vi "Log_ADAM_scan_table.vi"() -> ()   [LabVIEW 2015]
uses:
  ADAM Client/Sub VIs/ADAM Controls/Channel_State.ctl
  Anemometry/Anemometry Sub Vis/Globals/Constants_global.vi
  Anemometry/Anemometry Sub Vis/Globals/Preference_global.vi
  ADAM_Global.vi
  Anemometry/Anemometry Sub Vis/Globals/Meas_global.vi
panel:
  in  "High Res Day files":bool=TRUE
  in  "Ventilate Lab if temp above":dbl=21.5
  in  "Averaging time (Seconds)":dbl=60.0
  out "Current time":string
  out "Started Time":string
  in  "stop":bool
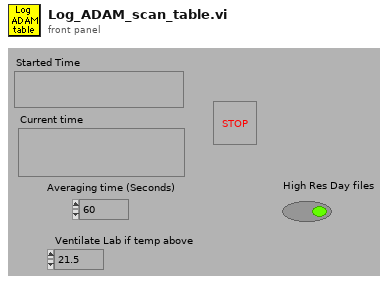
[diagram p1: front panel]
types:
  T1 = enum16{"On", "Off", "Always On", "Always Off", "Delete"}
  T2 = typedef "Channel_State.ctl" = enum16{"On", "Off", "Always On", "Always Off"}
  T3 = enum16{"Load ADAM setup from excel file", "Save ADAM setup to excel file"}
  T4 = cluster{"second":i32, "minute":i32, "hour":i32, "day of month":i32, "month":i32, "year":i32, "day of week":i32, "day of year":i32, "is DST":i32}
  T5 = typedef "Client_State_Cluster.ctl" = cluster{"Client Name":string, "Traverse level State":T6, "People to Email":string[], "Next Contact Time":dbl}
  T6 = typedef "Traverse_Level_State.ctl" = enum16{"Running", "Complete"}
  T7 = typedef "Server_Control.ctl" = cluster{"Channel Name to control":string, "Channel sharing":enum16{"Channel Unshared", "Channel Shared by Rig", "Channel Shared by Group"}, "Default Value":dbl, "Client Array":string[], "Time Stamp":timestamp, "Do Not Reset":bool}
  T8 = typedef "LVDateTimeRec.ctl" = cluster{"fractional second":dbl, "second":i32, "minute":i32, "hour":i32, "day of month":i32, "month":i32, "year":i32, "day of week":i32, "day of year":i32, "DST":i32}
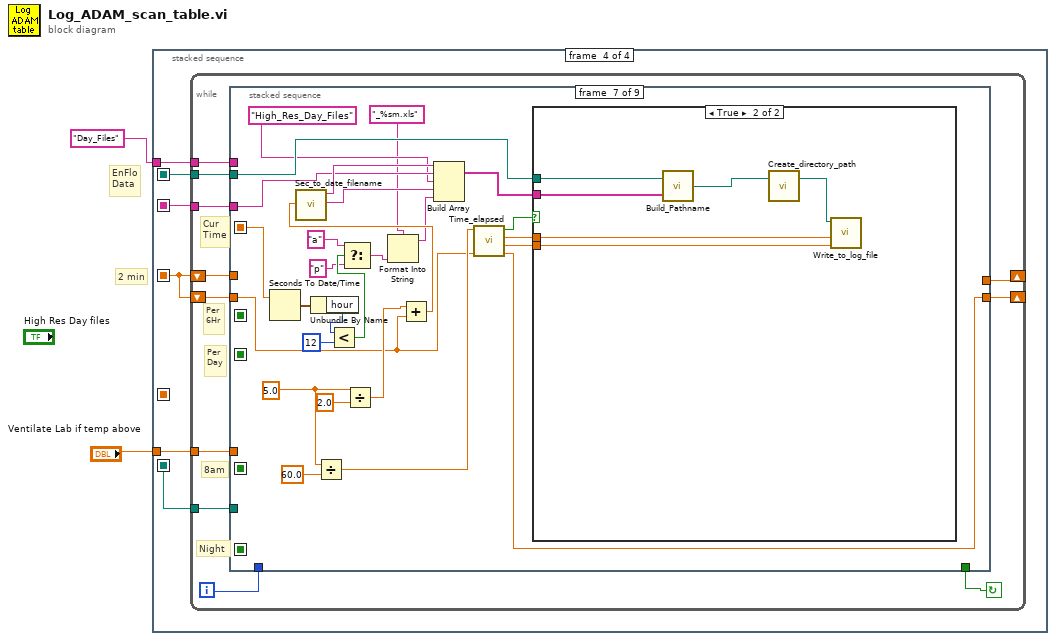
[diagram p0: block diagram]
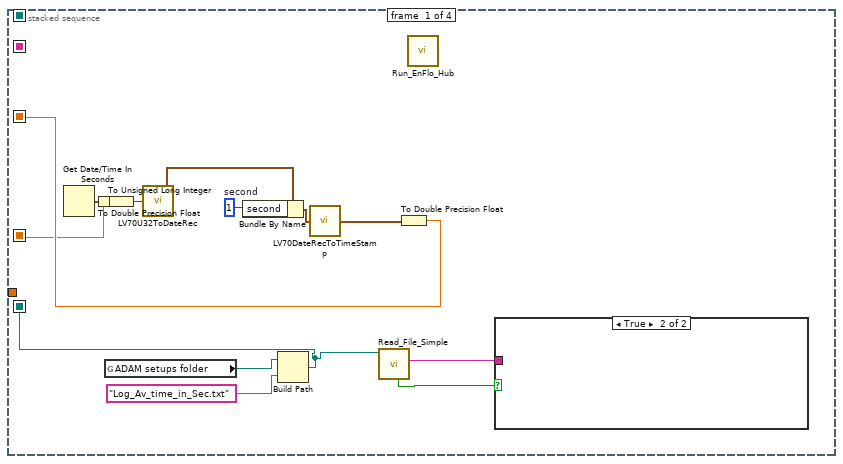
[diagram p2: hidden frame]
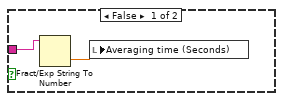
[diagram p3: hidden frame]
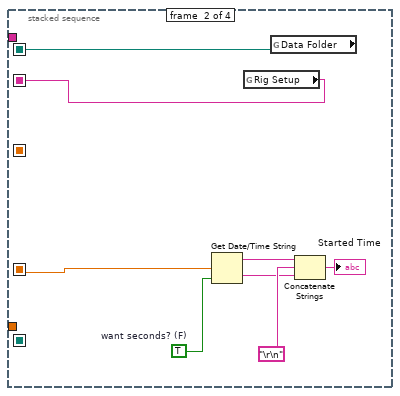
[diagram p4: hidden frame]
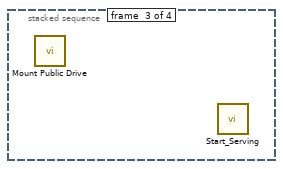
[diagram p5: hidden frame]
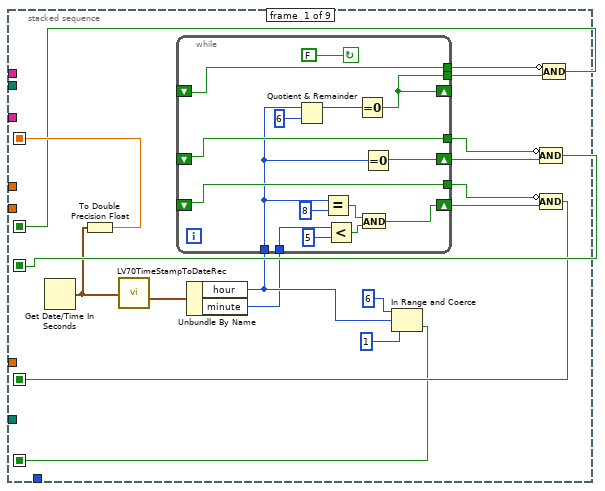
[diagram p6: hidden frame]
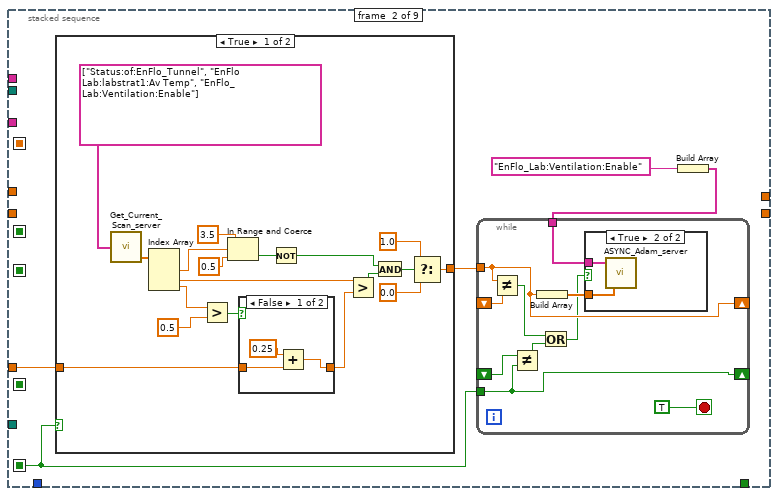
[diagram p7: hidden frame]
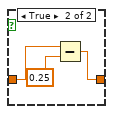
[diagram p9: hidden frame]
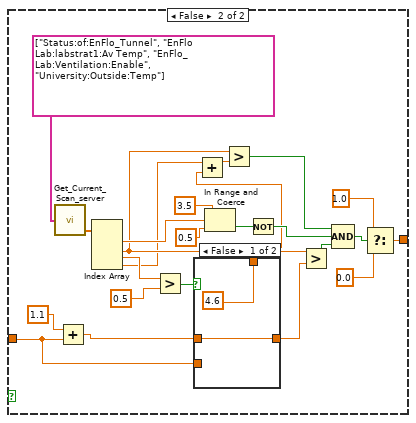
[diagram p10: hidden frame]
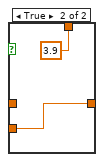
[diagram p11: hidden frame]
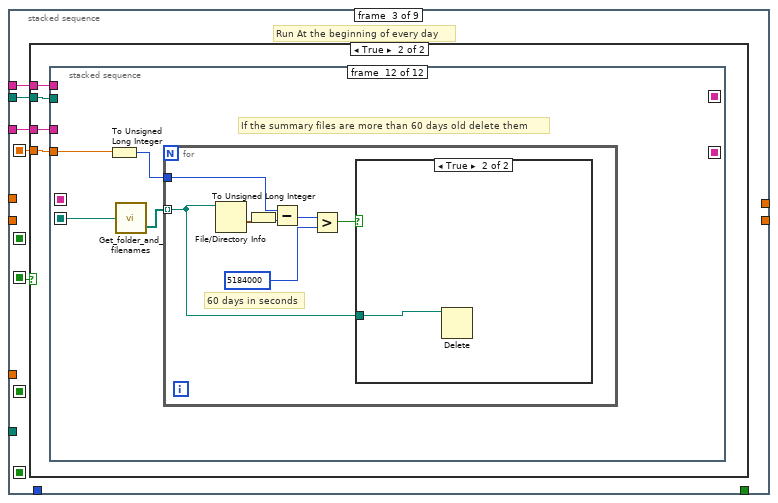
[diagram p12: hidden frame]
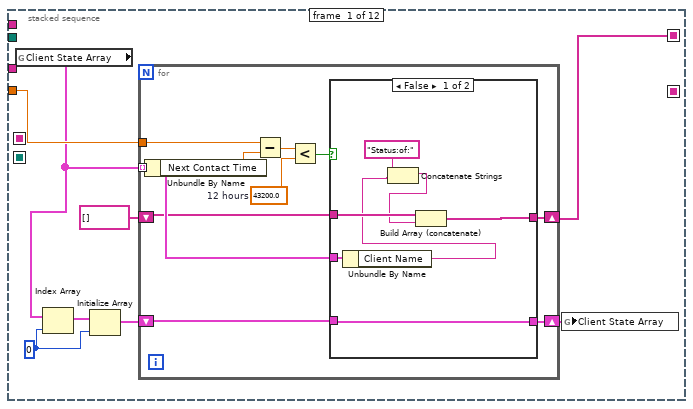
[diagram p14: hidden frame]
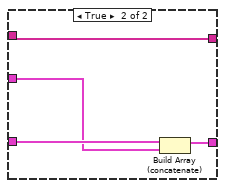
[diagram p15: hidden frame]
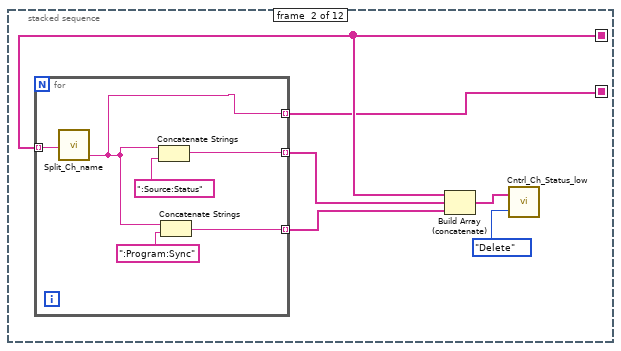
[diagram p16: hidden frame]
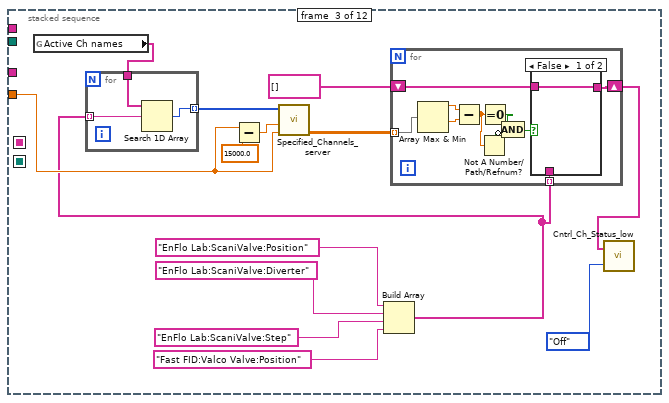
[diagram p17: hidden frame]
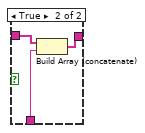
[diagram p18: hidden frame]
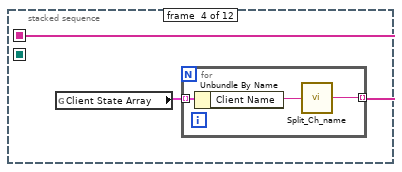
[diagram p19: hidden frame]
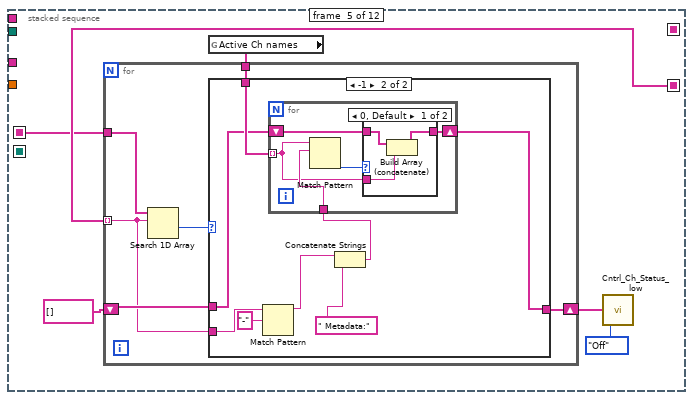
[diagram p20: hidden frame]
diagram:
  # "EnFlo\nData"
  # "2 min"
  n1 = stacked-sequence {
    seq-local: [w13 _ _ _] -> [_ _ _ w26]
    seq-local: [w12 _ _ _] -> [_ w25 _ _]
    seq-local: [_ w19 _ _] -> [_ _ _ w31]
    seq-local: [w5 _ _ _] -> [_ _ _ w29]
    seq-local: [_ w18 _ _] -> [_ _ _ w28]
    tunnel: "Day_Files" ("Input Element") -> [_ _ _ w30]
    tunnel: "Ventilate Lab if temp above" -> [_ _ _ w27]
    frame #0 {
      w15 = 1  # second
      n2 = Get Date/Time In Seconds() -> (seconds since 1Jan1904=w9:timestamp)
      n3 = To Double Precision Float(number=w9) -> (double precision float=w12:dbl)
      n4 = global read "Constants_global.vi" "ADAM setups folder"() -> (w7:path)
      n5 = To Unsigned Long Integer(number=w12) -> (unsigned 32bit integer=w11:u32)
      n6 = call <vilib>:"LV70U32ToDateRec.vi"("Time"=w11) -> ("date time rec"=w10:T4)
      n7 = Bundle By Name(cluster=w10, "second"=w15) -> (w14:T4)
      n8 = Build Path(base path=w7, name or relative path="Log_Av_time_in_Sec.txt") -> (appended path=w5:path)
      n9 = call <vilib>:"LV70DateRecToTimeStamp.vi"("date time rec"=w14) -> ("Time Stamp"=w8:timestamp)
      n10 = call "Read_File_Simple.vi"("Filename"=w5) -> ("Error?"=w3:bool, "string"=w4:string)  [unwired: 2 in, 6 out]
      n11 = To Double Precision Float(number=w8) -> (double precision float=w13:dbl)
      n12 = call "Run_EnFlo_Hub.vi"() -> ()  [unwired: 8 out]
      n13 = case shown="True" w3 {
        tunnel: w4 -> [w17 _]
        frame False {
          n14 = Fract/Exp String To Number(string=w17) -> (number=w16:dbl)  [unwired: 4 out]
          n15 = local write "Averaging time (Seconds)"(w16) -> ()
        }
        frame True {
        }
      }
    }
    frame #1 {
      w24 = TRUE  # want seconds? (F)
      n16 = Get Date/Time String(seconds (now)=w25, want seconds? (F)=w24) -> (date string=w22:string, time string=w21:string)  [unwired: 1 out]
      n17 = global read "Preference_global.vi" "Rig Setup"() -> (w18:string)
      n18 = global read "Constants_global.vi" "Data Folder"() -> (w19:path)
      n19 = Concatenate Strings(w22, "\r\n", w21) -> (→"Started Time":string)
    }
    frame #2 {
      n20 = call "Mount Public Drive.vi"() -> ()  [unwired: 12 in]
      n21 = call "Start_Serving.vi"() -> ()  [unwired: 1 out]
    }
    frame #3 {
      n22 = while {
        tunnel: w31 -> [w40]
        shift-left: w26 -> [w42]
        shift-right: [w41] -> _
        tunnel: w30 -> [w37]
        tunnel: w29 -> [w36]
        tunnel: w28 -> [w35]
        tunnel: w27 -> [w34]
        shift-right: [w32] -> _
        shift-left: w26 -> [w33]
        i -> [w39]
        stop <- w38 continue-if-true
        # "Night"
        # "8am"
        # "Per\n6Hr"
        # "Per\nDay"
        # "Cur\nTime"
        n23 = stacked-sequence {
          seq-local: [w52 _ _ _ _ _ _ _ _] -> [_ _ w148 _ _ _ _ _ _]
          seq-local: [w58 _ _ _ _ _ _ _ _] -> [_ _ w147 w374 w393 _ w433 _ _]
          seq-local: [w55 _ _ _ _ _ _ _ _] -> [_ _ _ _ _ _ _ _ _]
          seq-local: [w48 _ _ _ _ _ _ _ _] -> [_ _ _ w370 _ _ _ _ _]
          seq-local: [w44 _ _ _ _ _ _ _ _] -> [_ w75 _ _ _ _ _ _ _]
          tunnel: [_ _ _ _ _ w400 _ _ _] -> w41
          tunnel: w42 -> [_ _ _ _ _ w401 _ _ _]
          tunnel: w40 -> [_ _ w146 w373 _ w408 w448 _ _]
          tunnel: w39 -> [_ _ _ _ _ _ _ _ _]
          tunnel: [_ _ _ _ _ _ _ _ w468] -> w38
          tunnel: w37 -> [_ _ w145 w372 _ w398 _ _ _]
          tunnel: w36 -> [_ _ _ _ _ _ _ _ w467]
          tunnel: w35 -> [_ _ w144 w371 _ w402 w443 _ _]
          tunnel: w34 -> [_ w76 _ _ _ _ _ _ _]
          tunnel: w33 -> [_ _ _ _ _ _ w441 _ _]
          tunnel: [_ _ _ _ _ _ w440 _ _] -> w32
          frame #0 {
            n24 = Get Date/Time In Seconds() -> (seconds since 1Jan1904=w51:timestamp)
            n25 = To Double Precision Float(number=w51) -> (double precision float=w58:dbl)
            n26 = call <vilib>:"LV70TimeStampToDateRec.vi"("time stamp"=w51) -> ("date time rec"=w59:T4)
            n27 = Unbundle By Name(w59) -> ("hour"=w47:i32, "minute"=w43:i32)
            n28 = while {
              tunnel: [w69] -> w53
              shift-left: _ -> [w69]
              shift-right: [w70] -> w54
              tunnel: [w71] -> w56
              tunnel: [w72] -> w57
              tunnel: w47 -> [w66]
              shift-left: _ -> [w71]
              shift-right: [w72] -> _
              tunnel: [w67] -> w50
              shift-right: [w60] -> w49
              shift-left: _ -> [w67]
              tunnel: w43 -> [w64]
              stop <- FALSE continue-if-true
              n29 = Quotient & Remainder(x=w66, y=6) -> (x-y*floor(x/y)=w73:i32)  [unwired: 1 out]
              n30 = Equal?(x=w66, y=8) -> (x = y?=w61:bool)
              n31 = Less?(x=w64, y=5) -> (x < y?=w62:bool)
              n32 = Equal To 0?(x=w73) -> (x = 0?=w72:bool)
              n33 = And(x=w61, y=w62) -> (x .and. y?=w60:bool)
              n34 = Equal To 0?(x=w66) -> (x = 0?=w70:bool)
            }
            n35 = In Range and Coerce(upper limit=6, x=w47, lower limit=1) -> (In Range?=w44:bool)  [unwired: 1 out]
            n36 = Compound Arithmetic op=AND(invert w53, w54) -> (w52:bool)
            n37 = Compound Arithmetic op=AND(invert w50, w49) -> (w48:bool)
            n38 = Compound Arithmetic op=AND(invert w56, w57) -> (w55:bool)
          }
          frame #1 {
            n39 = case shown="True" w75 {
              tunnel: [w102 w133] -> w77
              tunnel: w76 -> [w92 w116]
              frame True {
                n40 = call "Get_Current_Scan_server.vi"("Desired Channels"=string[] ["Status:of:EnFlo_Tunnel", "EnFlo Lab:labstrat1:Av Temp", "EnFlo_Lab:Ventilation:Enable"]) -> ("Numerical Values"=w108:dbl[])  [unwired: 2 out]
                n41 = Index Array(array=w108) -> (element #1=w101:dbl, element #2=w107:dbl, element #3=w96:dbl)  [unwired: 3 in]
                n42 = Greater?(x=w96, y=0.5) -> (0:w94:bool)
                n43 = In Range and Coerce(upper limit=3.5, x=w101, lower limit=0.5) -> (In Range?=w98:bool)  [unwired: 1 out]
                n44 = case shown="False" w94 {
                  tunnel: [w111 w113] -> w93
                  tunnel: w92 -> [w112 w115]
                  frame False {
                    n45 = Add(x=0.25, y=w112) -> (x+y=w111:dbl)
                  }
                  frame True {
                    n46 = Subtract(x=w115, y=0.25) -> (x-y=w113:dbl)
                  }
                }
                n47 = Not(x=w98) -> (.not. x?=w97:bool)
                n48 = Greater?(x=w107, y=w93) -> (0:w106:bool)
                n49 = And(x=w97, y=w106) -> (x .and. y?=w105:bool)
                n50 = Select(t=1.0, s=w105, f=0.0) -> (s? t:f=w102:dbl)
              }
              frame False {
                n51 = call "Get_Current_Scan_server.vi"("Desired Channels"=string[] ["Status:of:EnFlo_Tunnel", "EnFlo Lab:labstrat1:Av Temp", "EnFlo_Lab:Ventilation:Enable", "University:Outside:Temp"]) -> ("Numerical Values"=w138:dbl[])  [unwired: 2 out]
                n52 = Add(x=1.1, y=w116) -> (x+y=w123:dbl)
                n53 = Index Array(array=w138) -> (element #1=w132:dbl, element #2=w121:dbl, element #3=w127:dbl, element #4=w120:dbl)  [unwired: 4 in]
                n54 = Greater?(x=w127, y=0.5) -> (0:w125:bool)
                n55 = case shown="False" w125 {
                  tunnel: [w141 w142] -> w124
                  tunnel: w123 -> [w141 _]
                  tunnel: [4.6 ("y") 3.9 ("y")] -> w117
                  tunnel: w116 -> [_ w142]
                  frame False {
                  }
                  frame True {
                  }
                }
                n56 = Add(x=w120, y=w117) -> (x+y=w119:dbl)
                n57 = In Range and Coerce(upper limit=3.5, x=w132, lower limit=0.5) -> (In Range?=w129:bool)  [unwired: 1 out]
                n58 = Greater?(x=w121, y=w119) -> (0:w118:bool)
                n59 = Not(x=w129) -> (.not. x?=w128:bool)
                n60 = Greater?(x=w121, y=w124) -> (0:w137:bool)
                n61 = Compound Arithmetic op=AND(w118, w128, w137) -> (w136:bool)
                n62 = Select(t=1.0, s=w136, f=0.0) -> (s? t:f=w133:dbl)
              }
            }
            n63 = Build Array("EnFlo_Lab:Ventilation:Enable") -> (w78:string[])
            n64 = while {
              shift-right: [w87] -> _
              shift-left: _ -> [w88]
              tunnel: w77 -> [w87]
              tunnel: w78 -> [w85]
              shift-right: [w84] -> _
              shift-left: _ -> [w83]
              tunnel: w75 -> [w84]
              stop <- TRUE stop-if-true
              n65 = Not Equal?(x=w87, y=w88) -> (x != y?=w81:bool)
              n66 = Not Equal?(x=w83, y=w84) -> (x != y?=w82:bool)
              n67 = Build Array(w87) -> (w89:dbl[])
              n68 = Or(x=w81, y=w82) -> (x .or. y?=w80:bool)
              n69 = case shown="True" w80 {
                tunnel: w89 -> [_ w91]
                tunnel: w85 -> [_ w90]
                frame False {
                }
                frame True {
                  n70 = call "ASYNC_Adam_server.vi"("Values"=w91, "Channel Names"=w90) -> ()  [unwired: 1 in, 3 out]
                }
              }
            }
          }
          frame #2 {
            # "Run At the beginning of every day"
            n71 = case shown="True" w148 {
              tunnel: w147 -> [_ w152]
              tunnel: w146 -> [_ w151]
              tunnel: w145 -> [_ w150]
              tunnel: w144 -> [_ w149]
              frame False {
              }
              frame True {
                n72 = stacked-sequence {
                  seq-local: [w153 _ _ _ _ _ _ _ _ _ _ _] -> [_ w187 _ _ _ _ _ _ w307 _ _ _]
                  seq-local: [_ w183 _ _ _ _ _ _ _ _ _ _] -> [_ _ _ _ w235 _ _ _ _ _ _ _]
                  seq-local: [_ _ _ w225 _ _ _ _ _ _ _ _] -> [_ _ _ _ w232 _ _ _ _ _ _ _]
                  seq-local: [_ _ _ _ _ _ _ _ _ _ w356 _] -> [_ _ _ _ _ _ _ _ _ _ _ w360]
                  tunnel: w152 -> [w160 _ w204 _ _ _ _ _ _ w354 _ w361]
                  tunnel: w151 -> [_ _ _ _ _ _ _ _ _ _ _ _]
                  tunnel: w150 -> [_ _ _ _ _ _ _ _ _ _ _ _]
                  tunnel: w149 -> [_ _ _ _ _ _ _ _ _ _ _ _]
                  frame #0 {
                    w158 = 0 ("Index")
                    n73 = global read "ADAM_Global.vi" "Client State Array"() -> (w159:T5[])
                    n74 = Index Array(array=w159, index=w158) -> (element=w157:T5)
                    n75 = Initialize Array(w157, w158) -> (w156:T5[])
                    n76 = for {
                      tunnel: w159 -> [w163] mode=indexing
                      shift-right: [w164] -> w155
                      shift-left: w156 -> [w165]
                      tunnel: w160 -> [w170]
                      shift-right: [w161] -> w153
                      shift-left: string[] [] -> [w162]
                      w167 = 43200.0  # 12 hours
                      n77 = Unbundle By Name(w163) -> ("Next Contact Time"=w169:dbl)
                      n78 = Subtract(x=w170, y=w169) -> (x-y=w168:dbl)
                      n79 = Less?(x=w168, y=w167) -> (x < y?=w166:bool)
                      n80 = case shown="False" w166 {
                        tunnel: w165 -> [w177 w181]
                        tunnel: [w177 w180] -> w164
                        tunnel: w163 -> [w176 w179]
                        tunnel: w162 -> [w175 w178]
                        tunnel: [w174 w178] -> w161
                        frame False {
                          n81 = Unbundle By Name(w176) -> ("Client Name"=w172:string)
                          n82 = Concatenate Strings("Status:of:", w172) -> (w171:string)
                          n83 = Build Array (concatenate)(w175, w171) -> (w174:string[])
                        }
                        frame True {
                          n84 = Build Array (concatenate)(w181, w179) -> (w180:T5[])
                        }
                      }
                    }
                    n85 = global write "ADAM_Global.vi" "Client State Array"(w155) -> ()
                  }
                  frame #1 {
                    n86 = for {
                      tunnel: w187 -> [w193] mode=indexing
                      tunnel: [w190] -> w185 mode=indexing
                      tunnel: [w189] -> w184 mode=indexing
                      tunnel: [w188] -> w183 mode=indexing
                      n87 = call "Split_Ch_name.vi"("Ch name"=w193) -> ("Low level"=w188:string)  [unwired: 2 out]
                      n88 = Concatenate Strings(w188, ":Source:Status") -> (w190:string)
                      n89 = Concatenate Strings(w188, ":Program:Sync") -> (w189:string)
                    }
                    n90 = Build Array (concatenate)(w187, w185, w184) -> (w186:string[])
                    n91 = call "Cntrl_Ch_Status_low.vi"("Mode"=T1."Delete", "Channel names"=w186) -> ()  [unwired: 1 out]
                  }
                  frame #2 {
                    n92 = global read "ADAM_Global.vi" "Active Ch names"() -> (w207:string[])
                    n93 = Subtract(x=w204, y=15000.0) -> (x-y=w202:dbl)
                    n94 = Build Array("EnFlo Lab:ScaniValve:Position", "EnFlo Lab:ScaniValve:Diverter", "EnFlo Lab:ScaniValve:Step", "Fast FID:Valco Valve:Position") -> (w200:string[])
                    n95 = for {
                      tunnel: w207 -> [w224]
                      tunnel: w200 -> [w223] mode=indexing
                      tunnel: [w222] -> w205 mode=indexing
                      n96 = Search 1D Array(1D array=w224, element=w223) -> (index of element=w222:i32)  [unwired: 1 out]
                    }
                    n97 = call "Specified_Channels_server.vi"("End time"=w204, "Start time"=w202, "Requested channels"=w205) -> ("Output array"=w201:dbl[][])  [unwired: 2 in, 4 out]
                    n98 = for {
                      tunnel: w201 -> [w214] mode=indexing
                      shift-right: [w215] -> w195
                      shift-left: string[] [] -> [w209]
                      tunnel: w200 -> [w210] mode=indexing
                      n99 = Array Max & Min(array=w214) -> (max value=w217:dbl, min value=w216:dbl)  [unwired: 2 out]
                      n100 = Subtract(x=w217, y=w216) -> (x-y=w213:dbl)
                      n101 = Not A Number/Path/Refnum?(number/path/refnum=w213) -> (NaN/Path/Refnum?=w211:bool)
                      n102 = Equal To 0?(x=w213) -> (x = 0?=w208:bool)
                      n103 = Compound Arithmetic op=AND(w208, invert w211) -> (w212:bool)
                      n104 = case shown="False" w212 {
                        tunnel: [w218 w221] -> w215
                        tunnel: w210 -> [_ w220]
                        tunnel: w209 -> [w218 w219]
                        frame False {
                        }
                        frame True {
                          n105 = Build Array (concatenate)(w219, w220) -> (w221:string[])
                        }
                      }
                    }
                    n106 = call "Cntrl_Ch_Status_low.vi"("Mode"=T1."Off", "Channel names"=w195) -> ()  [unwired: 1 out]
                  }
                  frame #3 {
                    n107 = global read "ADAM_Global.vi" "Client State Array"() -> (w226:T5[])
                    n108 = for {
                      tunnel: w226 -> [w229] mode=indexing
                      tunnel: [w227] -> w225 mode=indexing
                      n109 = Unbundle By Name(w229) -> ("Client Name"=w228:string)
                      n110 = call "Split_Ch_name.vi"("Ch name"=w228) -> ("Middle"=w227:string)  [unwired: 2 out]
                    }
                  }
                  frame #4 {
                    n111 = global read "ADAM_Global.vi" "Active Ch names"() -> (w233:string[])
                    n112 = for {
                      tunnel: w235 -> [w236] mode=indexing
                      shift-right: [w239] -> w231
                      shift-left: string[] [] -> [w240]
                      tunnel: w233 -> [w238]
                      tunnel: w232 -> [w237]
                      n113 = Search 1D Array(1D array=w237, element=w236) -> (index of element=w241:i32)  [unwired: 1 out]
                      n114 = case shown="-1" w241 {
                        tunnel: w240 -> [w242 w248]
                        tunnel: [w242 w247] -> w239
                        tunnel: w236 -> [_ w243]
                        tunnel: w238 -> [_ w249]
                        frame 0, Default {
                        }
                        frame -1 {
                          n115 = Match Pattern(string=w243, regular expression="-") -> (before substring=w244:string)  [unwired: 4 out]
                          n116 = Concatenate Strings(w244, " Metadata:" ("Substring")) -> (w246:string)
                          n117 = for {
                            shift-right: [w253] -> w247
                            shift-left: w248 -> [w254]
                            tunnel: w246 -> [w252]
                            tunnel: w249 -> [w251] mode=indexing
                            n118 = Match Pattern(string=w251, regular expression=w252) -> (offset past match=w255:i32)  [unwired: 4 out]
                            n119 = case shown="0, Default" w255 {
                              tunnel: w254 -> [w257 w259]
                              tunnel: [w256 w259] -> w253
                              tunnel: w251 -> [w258 _]
                              frame 0, Default {
                                n120 = Build Array (concatenate)(w257, w258) -> (w256:string[])
                              }
                              frame -1 {
                              }
                            }
                          }
                        }
                      }
                    }
                    n121 = call "Cntrl_Ch_Status_low.vi"("Mode"=T1."Off", "Channel names"=w231) -> ()  [unwired: 1 out]
                  }
                  frame #5 {
                    n122 = Build Array("EnFlo_Tunnel:Heater:Enable") -> (w265:string[])
                    n123 = call "Get_Current_Scan_server.vi"("Desired Channels"=w265) -> ("Numerical Values"=w264:dbl[])  [unwired: 2 out]
                    n124 = Index Array(array=w264, index=0) -> (element=w262:dbl)
                    n125 = Less?(x=w262, y=0.5) -> (x < y?=w260:bool)
                    n126 = case shown="True" w260 {
                      frame False {
                      }
                      frame True {
                        w271 = "EnFlo_Tunnel:Setpo"
                        n127 = global read "ADAM_Global.vi" "Active Ch names"() -> (w269:string[])
                        n128 = String Length(string=w271) -> (length=w270:i32)
                        n129 = for {
                          shift-right: [w279] -> w268
                          shift-left: string[] [] -> [w281]
                          tunnel: w269 -> [w280] mode=indexing
                          tunnel: w270 -> [w283]
                          tunnel: w271 -> [w282]
                          tunnel: "EnFlo_Tunnel:Power" -> [w277]
                          n130 = String Subset(string=w280, length (rest)=w283) -> (substring=w278:string)  [unwired: 1 out]
                          n131 = Equal?(x=w278, y=w282) -> (x = y?=w275:bool)
                          n132 = Equal?(x=w278, y=w277) -> (x = y?=w276:bool)
                          n133 = Or(x=w275, y=w276) -> (x .or. y?=w274:bool)
                          n134 = case shown="True" w274 {
                            tunnel: w281 -> [w284 w287]
                            tunnel: w280 -> [_ w286]
                            tunnel: [w284 w285] -> w279
                            frame False {
                            }
                            frame True {
                              n135 = Build Array (concatenate)(w287, w286) -> (w285:string[])
                            }
                          }
                        }
                        n136 = call "Adam_Ch_on_off.vi"("Ch State"=Channel_State."Off", "ADAM Ch Names"=w268) -> ()  [unwired: 1 out]
                      }
                    }
                  }
                  frame #6 {
                    n137 = call "Read_Write_ADAM_setup.vi"("Mode"=T3."Save ADAM setup to excel file") -> ()  [unwired: 4 out]
                  }
                  frame #7 {
                    w292 = 5400.0  # 1.5 Hrs in seconds
                    n138 = Build Array("GMU:Source:Meas Q", "GMU:Source:Est Time") -> (w299:string[])
                    n139 = call "Get_Current_Scan_server.vi"("Desired Channels"=w299) -> ("Numerical Values"=w294:dbl[])  [unwired: 2 out]
                    n140 = Index Array(array=w294, index=0 ("Index")) -> (element=w296:dbl)
                    n141 = Index Array(array=w294, index=1 ("Index")) -> (element=w293:dbl)
                    n142 = Less?(x=w296, y=0.01) -> (x < y?=w290:bool)
                    n143 = Greater?(x=w293, y=w292) -> (0:w291:bool)
                    n144 = And(x=w290, y=w291) -> (x .and. y?=w289:bool)
                    n145 = case shown="True" w289 {
                      frame False {
                      }
                      frame True {
                        w302 = FALSE  # Activate channels
                        w303 = enum16{"Channel Name", "Main Address"}."Channel Name" ("Control on")
                        n146 = call "Ch_Active_Control.vi"("Match"="GMU:", "Activate Channels?"=w302, "Control on"=w303) -> ()  [unwired: 1 in, 2 out]
                        n147 = call "Ch_Active_Control.vi"("Match"="source", "Activate Channels?"=w302, "Control on"=w303) -> ()  [unwired: 1 in, 2 out]
                      }
                    }
                  }
                  frame #8 {
                    w311 = 0 ("Index")
                    n148 = global read "ADAM_Global.vi" "Server Control Array"() -> (w308:T7[])
                    n149 = Index Array(array=w308, index=w311) -> (element=w310:T7)
                    n150 = Initialize Array(w310, w311) -> (w309:T7[])
                    n151 = for {
                      tunnel: w308 -> [w313] mode=indexing
                      shift-right: [w318] -> w306
                      shift-left: w309 -> [w319]
                      tunnel: w307 -> [w317]
                      n152 = Unbundle By Name(w313) -> ("Client Array"=w316:string[])
                      n153 = for {
                        tunnel: w317 -> [w324]
                        tunnel: w316 -> [w322] mode=indexing
                        shift-right: [w320] -> w312
                        shift-left: string[] [] -> [w321]
                        n154 = Search 1D Array(1D array=w324, element=w322) -> (index of element=w323:i32)  [unwired: 1 out]
                        n155 = case shown="0, Default" w323 {
                          tunnel: w322 -> [_ w328]
                          tunnel: w321 -> [w325 w327]
                          tunnel: [w325 w326] -> w320
                          frame 0, Default {
                          }
                          frame -1 {
                            n156 = Build Array (concatenate)(w327, w328) -> (w326:string[])
                          }
                        }
                      }
                      n157 = Array Size(array=w312) -> (size(s)=w314:i32)
                      n158 = case shown="0" w314 {
                        tunnel: w319 -> [w329 w333]
                        tunnel: [w329 w334] -> w318
                        tunnel: w313 -> [_ w332]
                        tunnel: w312 -> [_ w331]
                        frame 0 {
                        }
                        frame 1, Default {
                          n159 = Bundle By Name(cluster=w332, "Client Array"=w331) -> (w330:T7)
                          n160 = Build Array (concatenate)(w333, w330) -> (w334:T7[])
                        }
                      }
                    }
                    n161 = global write "ADAM_Global.vi" "Server Control Array"(w306) -> ()
                  }
                  frame #9 {
                    w342 = "\r\n"
                    n162 = global write "Meas_global.vi" "Start Time of experiment"(w354) -> ()
                    n163 = global read "Constants_global.vi" "ADAM setups folder"() -> (w345:path)
                    n164 = Build Path(base path=w345, name or relative path="Setup_Files") -> (appended path=w349:path)
                    n165 = Build Path(base path=w345, name or relative path="Hi_Tec_Calibs.xls") -> (appended path=w344:path)
                    n166 = Build Path(base path=w349, name or relative path="Selected_Filename.txt" ("Substring")) -> (appended path=w351:path)
                    n167 = call "Read_File_Simple.vi"("Filename"=w351) -> ("string"=w350:string)  [unwired: 2 in, 7 out]
                    n168 = Build Path(base path=w349, name or relative path=w350) -> (appended path=w348:path)
                    n169 = call "Read_File_Simple.vi"("Filename"=w344) -> ("string"=w343:string)  [unwired: 2 in, 7 out]
                    n170 = call "Read_File_Simple.vi"("Filename"=w348) -> ("string"=w347:string)  [unwired: 2 in, 7 out]
                    n171 = call "Get_mod_dates.vi"() -> ("Output string"=w341:string)  [unwired: 1 in, 4 out]
                    n172 = call "Create_Error_log_folders.vi"("Per Day Log File?"=TRUE, "Log Filename"="ADAM_Setups" ("Substring")) -> ("Server copy Location"=w335:path, "Local Log File"=w337:path)  [unwired: 1 in, 1 out]
                    n173 = Concatenate Strings(w347, w342, w343, w342, w341) -> (w338:string)
                    n174 = call "Write_File_Simple.vi"("character string"=w338, "file path"=w337) -> ("file path Out"=w336:path)  [unwired: 1 in, 1 out]
                    n175 = call "Updated_File_Copy.vi"("Target Path"=w335, "Source Path"=w336) -> ()  [unwired: 2 out]
                  }
                  frame #10 {
                    n176 = global read "Constants_global.vi" "Data Folder Local"() -> (w357:path)
                    n177 = Build Path(base path=w357, name or relative path="Results_Summary_files") -> (appended path=w356:path)
                  }
                  frame #11 {
                    # "If the summary files are more than 60 days old delete them"
                    n178 = To Unsigned Long Integer(number=w361) -> (unsigned 32bit integer=w358:u32)
                    n179 = call "Get_folder_and_filenames.vi"("file path (dialog if empty)"=w360) -> ("Files"=w359:path[])  [unwired: 1 out]
                    n180 = for {
                      tunnel: w359 -> [w363] mode=indexing
                      tunnel: w358 -> [w368]
                      # "60 days in seconds"
                      n181 = File/Directory Info(path=w363) -> (last mod=w362:timestamp)  [unwired: 1 in, 6 out]
                      n182 = To Unsigned Long Integer(number=w362) -> (unsigned 32bit integer=w367:u32)
                      n183 = Subtract(x=w368, y=w367) -> (x-y=w366:u32)
                      n184 = Greater?(x=w366, y=u32 5184000) -> (0:w364:bool)
                      n185 = case shown="True" w364 {
                        tunnel: w363 -> [_ w369]
                        frame False {
                        }
                        frame True {
                          n186 = Delete(path (use dialog)=w369) -> ()  [unwired: 1 in, 6 out]
                        }
                      }
                    }
                  }
                }
              }
            }
          }
          frame #3 {
            # "At 8am every day"
            n187 = case shown="True" w370 {
              tunnel: w374 -> [_ w378]
              tunnel: w373 -> [_ w377]
              tunnel: w372 -> [_ w376]
              tunnel: w371 -> [_ w375]
              frame False {
              }
              frame True {
                n188 = stacked-sequence {
                  seq-local: [w386 _] -> [_ w392]
                  tunnel: w378 -> [w390 _]
                  tunnel: w377 -> [w379 _]
                  tunnel: w376 -> [w384 _]
                  tunnel: w375 -> [w380 _]
                  frame #0 {
                    n189 = Subtract(x=w390, y=36000.0) -> (x-y=w388:dbl)
                    n190 = call "Sec_to_date_filename.vi"("seconds"=w388) -> ("Year"=w385:string, "Month"=w389:string, "Day"=w382:string)  [unwired: 1 out]
                    n191 = Concatenate Strings(w382, ".xls" ("string")) -> (w381:string)
                    n192 = Build Array(w385, w380, w384, w389, w381) -> (w387:string[])
                    n193 = call "Build_Pathname.vi"("PathElements"=w387, "PathnameIn"=w379) -> ("AppendedPath"=w386:path)
                  }
                  frame #1 {
                    # "This VI emails a summary of all the server errors that occured Yesterday"
                    n194 = call "Adam_server_messages.vi"("Filename"=w392) -> ()  [unwired: 1 out]
                  }
                }
              }
            }
          }
          frame #4 {
            n195 = call "EnFlo_Seeder_Control.vi"("Current Time (s)"=w393) -> ()
            n196 = Wait (ms)(milliseconds to wait=u32 1000 ("milliseconds to Wait")) -> ()  [unwired: 1 out]
          }
          frame #5 {
            n197 = Divide(x="Averaging time (Seconds)", y=60.0) -> (x/y=w406:dbl)
            n198 = Divide(x="Averaging time (Seconds)", y=2.0) -> (x/y=w403:dbl)
            n199 = Add(x=w403, y=w401) -> (x+y=w399:dbl)
            n200 = call "Sec_to_date_filename.vi"("seconds"=w399) -> ("Year"=w410:string, "Month"=w411:string, "Time"=w396:string)  [unwired: 1 out]
            n201 = Concatenate Strings(w396, ".xls" ("string")) -> (w397:string)
            n202 = Build Array(w410, w402, w398, w411, w397) -> (w409:string[])
            n203 = call "Time_elapsed.vi"("End of previous average in"=w401, "Averaging time (mins)"=w406) -> ("End of previous average out"=w400:dbl, "End of period"=w413:dbl, "Start of period"=w414:dbl, "Time elapsed ?"=w412:bool)  [unwired: 2 in]
            n204 = case shown="True" w412 {
              tunnel: w413 -> [_ w417]
              tunnel: w414 -> [_ w418]
              tunnel: w408 -> [_ w416]
              tunnel: w409 -> [_ w415]
              frame False {
              }
              frame True {
                n205 = stacked-sequence {
                  tunnel: w418 -> [w427 _]
                  tunnel: w417 -> [w426 _]
                  tunnel: w416 -> [w419 _]
                  tunnel: w415 -> [w422 _]
                  frame #0 {
                    n206 = global read "ADAM_Global.vi" "2 Min average comment"() -> (w425:string)
                    n207 = global read "Meas_global.vi" "Error Messages"() -> (w424:string)
                    n208 = call "Build_Pathname.vi"("PathElements"=w422, "PathnameIn"=w419) -> ("AppendedPath"=w421:path)
                    n209 = call "Create_directory_path.vi"("Path name"=w421) -> ("Path name Out"=w420:path)  [unwired: 1 in, 1 out]
                    n210 = Concatenate Strings(w425, w424) -> (w423:string)
                    n211 = call "Write_to_log_file.vi"("User added comment"=w423, "End time"=w426, "Start time"=w427, "Folder/file"=w420) -> ()  [unwired: 5 in, 3 out]
                  }
                  frame #1 {
                    w428 = ""
                    n212 = global write "ADAM_Global.vi" "2 Min average comment"(w428) -> ()
                    n213 = global write "Meas_global.vi" "Error Messages"(w428) -> ()
                  }
                }
              }
            }
          }
          frame #6 {
            w442 = 5.0 ("y")
            n214 = Seconds To Date/Time(time stamp (now)=w433) -> (date time rec=w439:T8)  [unwired: 1 in]
            n215 = Unbundle By Name(w439) -> ("hour"=w438:i32)
            n216 = Divide(x=w442, y=60.0) -> (x/y=w446:dbl)
            n217 = Less?(x=w438, y=12) -> (x < y?=w436:bool)
            n218 = Select(t="a", s=w436, f="p") -> (s? t:f=w432:string)
            n219 = Divide(x=w442, y=2.0) -> (x/y=w444:dbl)
            n220 = Format Into String(format string="_%sm.xls", w432) -> (resulting string=w429:string)  [unwired: 2 in, 1 out]
            n221 = Add(x=w444, y=w441) -> (x+y=w455:dbl)
            n222 = call "Sec_to_date_filename.vi"("seconds"=w455) -> ("Year"=w450:string, "Month"=w451:string)  [unwired: 2 out]
            n223 = Build Array(w450, w443, "High_Res_Day_Files" ("Input Element"), w451, w429) -> (w449:string[])
            n224 = call "Time_elapsed.vi"("End of previous average in"=w441, "Averaging time (mins)"=w446) -> ("End of previous average out"=w440:dbl, "End of period"=w453:dbl, "Start of period"=w454:dbl, "Time elapsed ?"=w452:bool)  [unwired: 2 in]
            n225 = case shown="True" w452 {
              tunnel: w453 -> [_ w460]
              tunnel: w454 -> [_ w461]
              tunnel: w448 -> [_ w459]
              tunnel: w449 -> [_ w458]
              frame False {
              }
              frame True {
                n226 = call "Build_Pathname.vi"("PathElements"=w458, "PathnameIn"=w459) -> ("AppendedPath"=w457:path)
                n227 = call "Create_directory_path.vi"("Path name"=w457) -> ("Path name Out"=w456:path)  [unwired: 1 in, 1 out]
                n228 = call "Write_to_log_file.vi"("End time"=w460, "Start time"=w461, "Folder/file"=w456) -> ()  [unwired: 6 in, 3 out]
              }
            }
          }
          frame #7 {
            w466 = TRUE  # want seconds? (F)
            n229 = Get Date/Time String(want seconds? (F)=w466) -> (date string=w464:string, time string=w463:string)  [unwired: 2 out]
            n230 = Concatenate Strings(w464, "\r\n", w463) -> (→"Current time":string)
          }
          frame #8 {
            n231 = while {
              shift-right: [w470] -> _
              shift-left: _ -> [w474]
              tunnel: w467 -> [w471]
              stop <- TRUE stop-if-true
              n232 = local read "Averaging time (Seconds)"() -> (w470:dbl)
              n233 = Not Equal?(x=w470, y=w474) -> (x != y?=w472:bool)
              n234 = case shown="True" w472 {
                tunnel: w471 -> [_ w475]
                tunnel: w470 -> [_ w477]
                frame False {
                }
                frame True {
                  n235 = Number To Fractional String(number=w477, precision (6)=i16 6) -> (F-format string=w476:string)  [unwired: 2 out]
                  n236 = call "Write_File_Simple.vi"("character string"=w476, "file path"=w475) -> ()  [unwired: 1 in, 2 out]
                }
              }
            }
            n237 = Not(x="stop") -> (.not. x?=w468:bool)
          }
        }
      }
    }
  }
